vi "test_udp2port.vi"() -> ()   [LabVIEW 2017]
panel:
  out "Numeric 2":i32
  out "data out":string
  in  "Stop":bool
  out "Numeric":i32
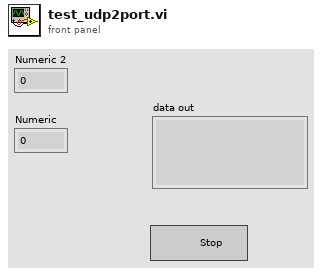
[diagram p1: front panel]
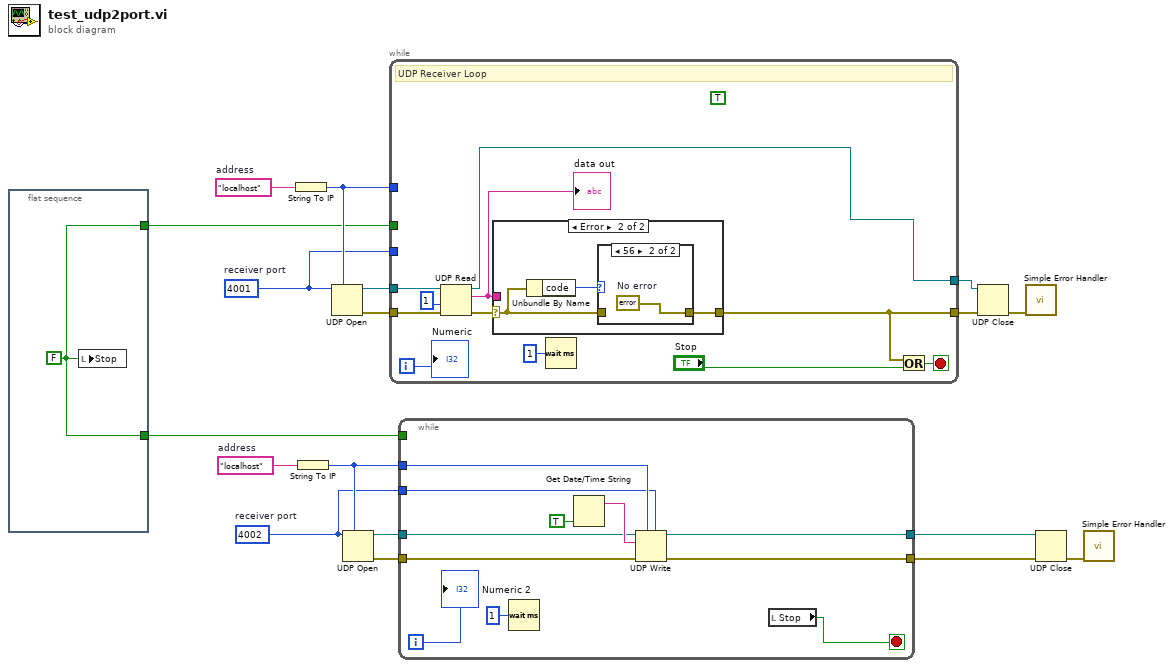
[diagram p0: block diagram]
diagram:
  w7 = "localhost"  # address
  w2 = u16 4002  # receiver port
  w14 = "localhost"  # address
  w1 = u16 4001  # receiver port
  n1 = flat-sequence {
    tunnel: [w19] -> w4
    tunnel: [w19] -> w3
    frame #0 {
      w19 = FALSE ("Stop")
      n2 = local write "Stop"(w19) -> ()
    }
  }
  n3 = String To IP(1:w14) -> (0:w13:u32)
  n4 = String To IP(1:w7) -> (0:w6:u32)
  n5 = UDP Open(7:w13, 11:w1) -> (port=w15:refnum<k16>, 0:w16:errorcluster)  [unwired: 3 in, 1 out]
  n6 = UDP Open(7:w6, 11:w2) -> (port=w11:refnum<k16>, 0:w12:errorcluster)  [unwired: 3 in, 1 out]
  n7 = while {
    tunnel: w15 -> [w30]
    tunnel: w16 -> [w27]
    tunnel: [w23] -> w17
    tunnel: w13 -> [_]
    tunnel: [w20] -> w5
    tunnel: w4 -> [_]
    tunnel: w1 -> [_]
    i -> [w24]
    stop <- w28 stop-if-true
    (unwired) TRUE ("want seconds? (F)")
    # "UDP Receiver Loop"
    n8 = UDP Read(connection ID=w30, timeout ms (25000)=1, 8:w27) -> (data out=w21:string, error out=w25:errorcluster, 3:w20:refnum<k16>)  [unwired: 3 out]
    "data out" <- w21
    n9 = case shown="Error" w25 {
      selector: w25 -> [w31 w33]
      tunnel: w21 -> [_ _]
      tunnel: [w31 w32] -> w23
      frame No Error {
        # "Sender sent data. Update the chart value."
      }
      frame Error {
        # "Sender did not send data. Ignore timeout error and keep waiting."
        n10 = Unbundle By Name(w33) -> ("code"=w34:i32)
        n11 = case shown="56" w34 {
          tunnel: w33 -> [w35 _]
          tunnel: [w35 w36] -> w32
          frame Default {
          }
          frame 56 {
            w36 = errorcluster {"status"=FALSE, "code"=0, "source"=""}  # No error
          }
        }
      }
    }
    n12 = Wait (ms)(milliseconds to wait=u32 1) -> ()  [unwired: 1 out]
    n13 = Or(x=w23, y="Stop") -> (x .or. y?=w28:bool)
    "Numeric" <- w24
  }
  n14 = while {
    tunnel: w12 -> [w44]
    tunnel: w11 -> [w43]
    tunnel: [w42] -> w9
    tunnel: [w41] -> w8
    tunnel: w6 -> [w40]
    tunnel: w3 -> [_]
    tunnel: w2 -> [w38]
    i -> [w39]
    stop <- w47 stop-if-true
    n15 = Wait (ms)(milliseconds to wait=u32 1) -> ()  [unwired: 1 out]
    n16 = Get Date/Time String(want seconds? (F)=TRUE) -> (time string=w45:string)  [unwired: 2 in, 1 out]
    n17 = UDP Write(address=w40, port or service name=w38, connection ID=w43, data in=w45, 8:w44) -> (error out=w42:errorcluster, 3:w41:refnum<k16>)  [unwired: 1 in]
    n18 = local read "Stop"() -> (w47:bool)
    "Numeric 2" <- w39
  }
  n19 = UDP Close(connection ID=w5, 8:w17) -> (error out=w18:errorcluster)  [unwired: 1 out]
  n20 = call <vilib>:"Simple Error Handler.vi"("error in (no error)"=w18) -> ()  [unwired: 1 in, 8 out]
  n21 = UDP Close(connection ID=w8, 8:w9) -> (error out=w10:errorcluster)  [unwired: 1 out]
  n22 = call <vilib>:"Simple Error Handler.vi"("error in (no error)"=w10) -> ()  [unwired: 1 in, 8 out]
